vi "Load INI file.vi"(8 "error in (no error)":errorcluster, 11 "Father of all uServices in":refnum<class "Father of all uServices.lvclass">) -> (0 "error out":errorcluster, 3 "Father of all uServices out":refnum<class "Father of all uServices.lvclass">)   [LabVIEW 2026, in "TALOS.lvlib" / "Father of all uServices.lvlib" / "Father of all uServices.lvclass"]
uses:
  Father of all uServices.lvclass
  Father of all uServices.lvclass/Father of all uServices.ctl
  Classes/Config/Config.lvclass
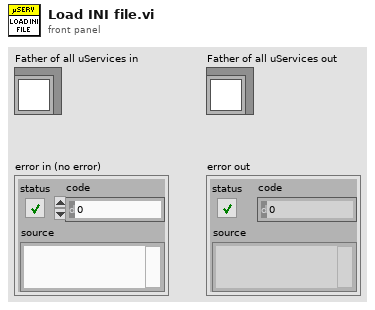
[diagram p1: front panel]
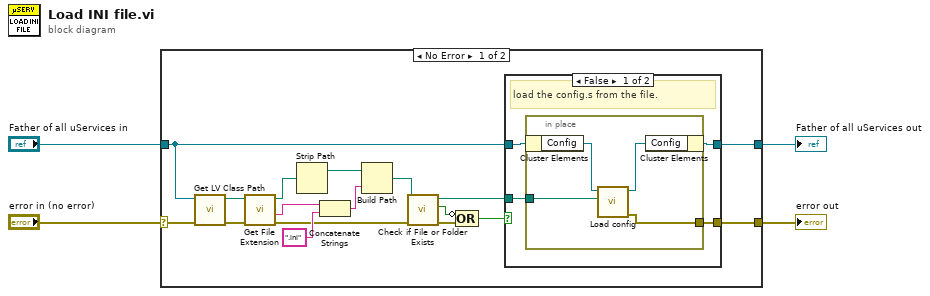
[diagram p0: block diagram]
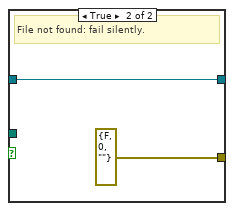
[diagram p2: hidden frame]
diagram:
  n1 = case shown="No Error" "error in (no error)" {
    selector: "error in (no error)" -> [w21 w33]
    tunnel: "Father of all uServices in" -> [w8 w32]
    tunnel: [w6 w33] -> w2
    tunnel: [w7 w32] -> w1
    frame No Error {
      n2 = call <vilib>:"Get LV Class Path.vi"("error in (no error)"=w21, "object"=w8) -> ("error out"=w19:errorcluster, "class path"=w20:path)  [unwired: 8 in]
      n3 = call <vilib>:"Get File Extension.vi"("error in (no error)"=w19, "file"=w20) -> ("error out"=w12:errorcluster, "filename without extension"=w15:string, "dup file"=w17:path)  [unwired: 5 in, 2 out]
      n4 = Strip Path(path=w17) -> (stripped path=w16:path)  [unwired: 1 out]
      n5 = Concatenate Strings(w15, ".ini" ("string")) -> (w18:string)
      n6 = Build Path(base path=w16, name or relative path=w18) -> (appended path=w13:path)
      n7 = call <vilib>:"Check if File or Folder Exists.vi"("error in (no error)"=w12, "path"=w13) -> ("error out"=w10:errorcluster, "file or folder exists?"=w11:bool, "dup path"=w5:path)  [unwired: 7 in]
      n8 = Compound Arithmetic op=OR(invert w11, w10) -> (w9:bool)
      n9 = case shown="False" w9 {
        tunnel: w8 -> [w24 w31]
        tunnel: [w23 w31] -> w7
        tunnel: [w22 errorcluster {"status"=FALSE, "code"=0, "source"=""} ("error constant")] -> w6
        tunnel: w5 -> [w25 _]
        frame False {
          # "load the config.s from the file."
          n10 = in-place {
            in-place-border: w25 -> [w27]
            in-place-border: [w26] -> w22
            n11 = in-place-cluster #1(w24) -> ("Config"=w29:refnum<class "Config.lvclass">)
            n12 = call "Load config.vi"("config file path"=w27, "Config in"=w29) -> ("error out"=w26:errorcluster, "Config out"=w28:refnum<class "Config.lvclass">)  [unwired: 8 in]
            n13 = in-place-cluster #1("Config"=w28) -> (w23:refnum<class "Father of all uServices.lvclass">)
          }
        }
        frame True {
          # "File not found: fail silently."
        }
      }
    }
    frame Error {
    }
  }
  "error out" <- w2
  "Father of all uServices out" <- w1
